vi "Test BitFile Parsing.vi"() -> ()   [LabVIEW 2011]
uses:
  <userlib>/_FPGA Interface Advanced Tools/FPGA Bitfile Utility/TypeDefs/Scalar Register Set.ctl
  <userlib>/_FPGA Interface Advanced Tools/FPGA Bitfile Utility/TypeDefs/Scalar Register.ctl
  TypeDefs/xVDT.ctl
  <userlib>/_FPGA Interface Advanced Tools/FPGA Bitfile Utility/FPGA Bitfile Utility.lvlib
  Sensor Simulation Custom Device.lvlib
panel:
  out "Resolvers":T1[](array[typedef])
  out "xVDTs":T1[](array[typedef])
  out "Control Scalars":T2
  out "error out":errorcluster
  in  "file path (use dialog)":path
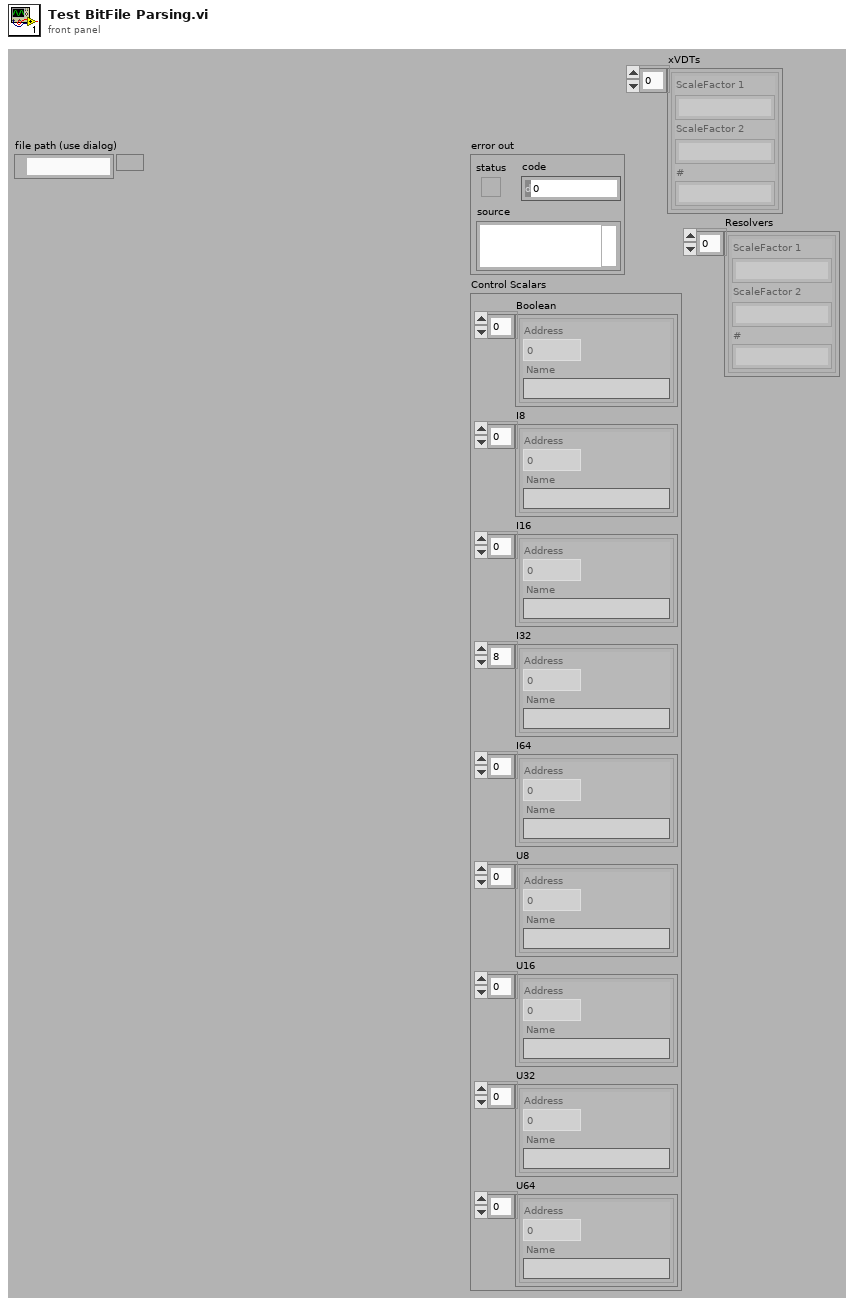
[diagram p1: front panel]
types:
  T1 = typedef "Sensor Simulation Custom Device.lvlib/xVDT.ctl" = cluster{"ScaleFactor 1":string, "ScaleFactor 2":string, "#":string}
  T2 = typedef "FPGA Bitfile Utility.lvlib/Scalar Register Set.ctl" = cluster{"Boolean":T3[], "I8":T3[], "I16":T3[], "I32":T3[], "I64":T3[], "U8":T3[], "U16":T3[], "U32":T3[], "U64":T3[]}
  T3 = typedef "FPGA Bitfile Utility.lvlib/Scalar Register.ctl" = cluster{"Address":u32, "Name":string}
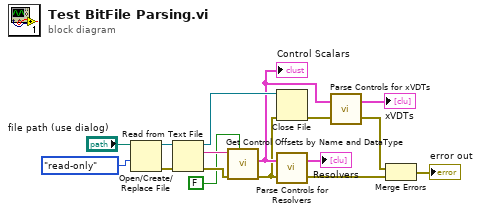
[diagram p0: block diagram]
diagram:
  n1 = Open/Create/Replace File(file path (use dialog)="file path (use dialog)", access (0:read/write)=enum16{"read/write", "read-only", "write-only"}."read-only") -> (refnum out=w12:refnum<file>, error out=w14:errorcluster)  [unwired: 4 in, 1 out]
  n2 = Read from Text File(file (use dialog)=w12, error in=w14) -> (refnum out=w10:refnum<file>, text=w11:string, error out=w13:errorcluster)  [unwired: 2 in, 1 out]
  n3 = call <userlib>:"Get Control Offsets by Name and DataType.vi"("User Specified?"=FALSE, "error in"=w13, "bitfile xml in"=w11) -> ("error out"=w4:errorcluster, "Control Scalars"=w5:T2)  [unwired: 3 in, 4 out]
  "Control Scalars" <- w5
  n4 = Close File(refnum=w10, error in=w4) -> (error out=w6:errorcluster)  [unwired: 1 out]
  n5 = call "Parse Controls for Resolvers.vi"("error in (no error)"=w4, "Control Scalars"=w5) -> ("error out"=w2:errorcluster, "Resolvers"=→"Resolvers":T1[])
  n6 = call "Parse Controls for xVDTs.vi"("error in (no error)"=w6, "Control Scalars"=w5) -> ("error out"=w3:errorcluster, "xVDTs"=→"xVDTs":T1[])
  n7 = Merge Errors(w3, w2) -> (→"error out":errorcluster)
